vi "Set Motor Modes 2017.vi"(7 "Robot Commands":T1) -> ()   [LabVIEW 2016]
uses:
  Drive and Climb SS/Drive + Climb Commands 2017.ctl
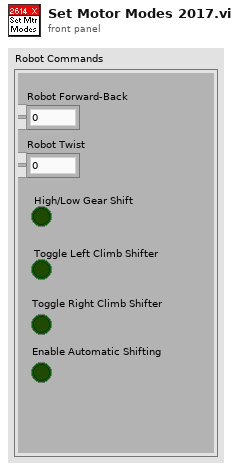
[diagram p1: front panel]
types:
  T1 = typedef "Drive + Climb Commands 2017.ctl" = cluster{"Robot Forward-Back":dbl, "Robot Twist":dbl, "High/Low Gear Shift":bool, "Toggle Left Climb Shifter":bool, "Toggle Right Climb Shifter":bool, "Enable Automatic Shifting":bool}
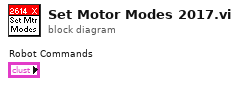
[diagram p0: block diagram]
diagram:
